vi "Configfile test.vi"() -> ()   [LabVIEW 2019]
uses:
  <vilib>/Utility/config.llb/Read Key (String).vi
  <vilib>/Utility/config.llb/Read Key (Double).vi
  <vilib>/Utility/config.llb/NI_LVConfig.lvlib
panel:
  out "found?":bool
  out "error out":errorcluster
  in  "configuration file path":path=path "E:/PHD/STF03/STF_Labview/Test.ini"
  out "Cluster":cluster{"String":string, "Numeric":dbl}
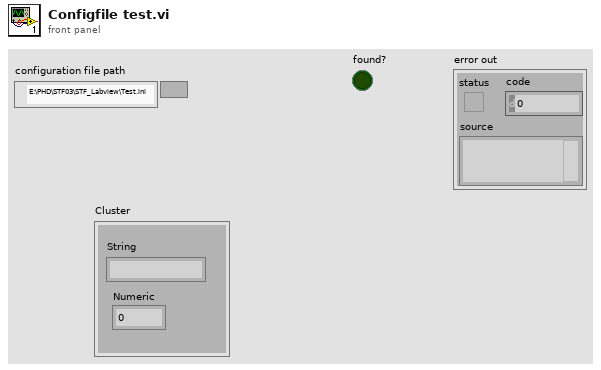
[diagram p1: front panel]
types:
  T1 = typedef "NI_LVConfig.lvlib/Config Data RefNum.ctl" = refnum<k1>
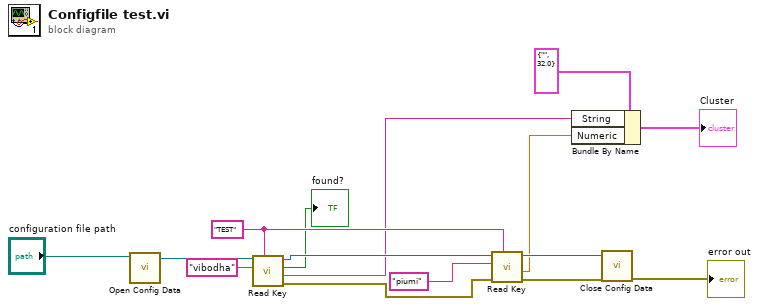
[diagram p0: block diagram]
diagram:
  w12 = "TEST" ("section")
  n1 = call <vilib>:"Open Config Data.vi"("configuration file path"="configuration file path") -> ("refnum"=w14:T1)  [unwired: 8 in, 2 out]
  n2 = call-poly <vilib>:"Read Key.vi"("section"=w12, "key"="vibodha", "refnum"=w14) -> ("error out"=w9:errorcluster, "value"=w5:string, "found?"=→"found?":bool, "refnum out"=w13:T1)  [unwired: 5 in]
  n3 = call-poly <vilib>:"Read Key.vi"("section"=w12, "error in (no error)"=w9, "key"="piumi", "refnum"=w13) -> ("error out"=w3:errorcluster, "value"=w1:dbl, "refnum out"=w4:T1)  [unwired: 4 in, 1 out]
  n4 = Bundle By Name(cluster=cluster{"String":string, "Numeric":dbl} {"String"="", "Numeric"=32.0} ("Cluster"), "String"=w5, "Numeric"=w1) -> (→"Cluster":cluster{"String":string, "Numeric":dbl})
  n5 = call <vilib>:"Close Config Data.vi"("error in (no error)"=w3, "refnum"=w4) -> ("error out"=→"error out":errorcluster)  [unwired: 8 in, 1 out]
